vi "Get Alicat Data.vi"(8 "error in":errorcluster, 11 "cCRDS Data in":refnum<class "cCRDS Data.lvclass">=refnum) -> (0 "error out":errorcluster, 2 "acData":T1(array[cluster]), 3 "cCRDS Data out":refnum<class "cCRDS Data.lvclass">)   [LabVIEW 2015, in "cCRDS Data.lvclass"]
uses:
  cCRDS Data.lvclass
  Devices/Alicat/Session Based/Data/Alicat Data.lvclass
  cCRDS Data.lvclass/cCRDS Data.ctl
  Read Serial Data.vi
  Reusable/Data/Data.lvclass
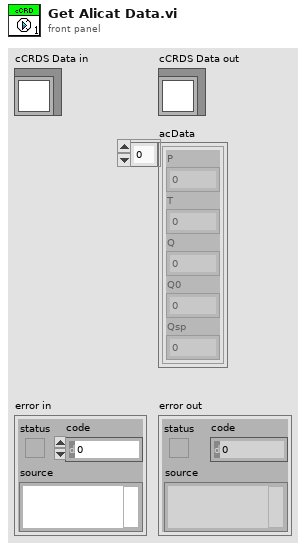
[diagram p1: front panel]
types:
  T1 = cluster{"P":sgl, "T":sgl, "Q":sgl, "Q0":sgl, "Qsp":sgl}[]
  T2 = cluster{"Accessors:Data[0]":sgl, "Accessors:Data[1]":sgl, "Accessors:Data[2]":sgl, "Accessors:Data[3]":sgl, "Accessors:Data[4]":sgl}
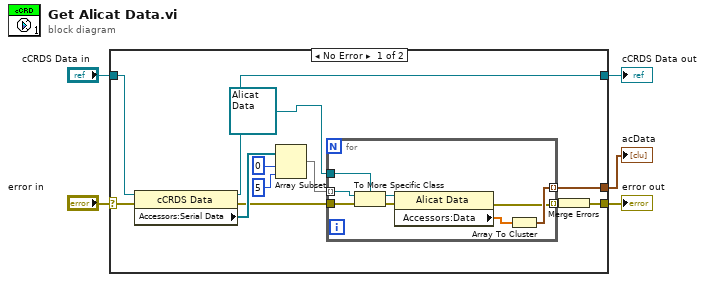
[diagram p0: block diagram]
diagram:
  n1 = case shown="No Error" "error in" {
    selector: "error in" -> [w16 w27]
    tunnel: [w8 w27] -> w4
    tunnel: [w15 w26] -> w2
    tunnel: "cCRDS Data in" -> [w17 w26]
    tunnel: [w7 _] -> w1
    frame No Error {
      n2 = property class="cCRDS Data"(reference=w17, error in=w16) -> (reference out=w15:refnum<class "cCRDS Data.lvclass">, error out=w10:errorcluster, "Accessors:Serial Data"=w14:refnum<class "Data.lvclass">[])
      n3 = Array Subset(array=w14, index=0, length=5) -> (w11:refnum<class "Data.lvclass">[])
      n4 = for {
        tunnel: w11 -> [w25] mode=indexing
        tunnel: refnum<class "Alicat Data.lvclass"> refnum ("Alicat Data") -> [w24]
        tunnel: w10 -> [w23]
        tunnel: [w18] -> w9 mode=indexing
        tunnel: [w19] -> w7 mode=indexing
        n5 = To More Specific Class(target class=w24, reference=w25, error in=w23) -> (specific class reference=w22:refnum<class "Alicat Data.lvclass">, error out=w21:errorcluster)
        n6 = property class="Alicat Data"(reference=w22, error in=w21) -> (error out=w18:errorcluster, "Accessors:Data"=w20:sgl[])  [unwired: 1 out]
        n7 = Array To Cluster(array=w20) -> (cluster=w19:T2)
      }
      n8 = Merge Errors(w9) -> (w8:errorcluster)
    }
    frame Error {
    }
  }
  "error out" <- w4
  "cCRDS Data out" <- w2
  "acData" <- w1
